vi "Ejercicio_6_Queued.vi"() -> ()   [LabVIEW 2020]
panel:
  out "Waveform Chart":dbl(graph)
  in  "stop":bool
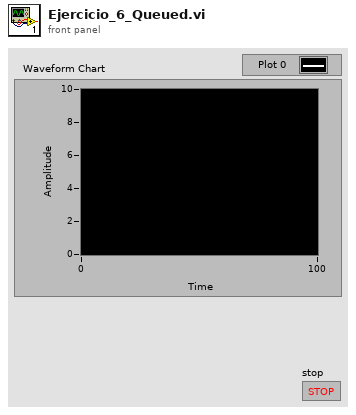
[diagram p1: front panel]
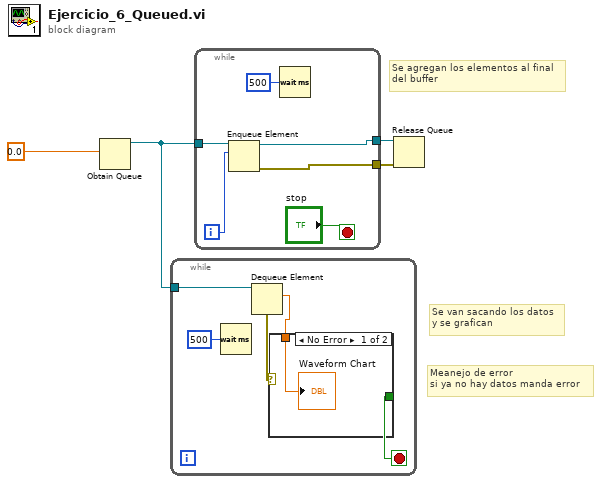
[diagram p0: block diagram]
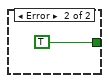
[diagram p2: hidden frame]
diagram:
  # "Se agregan los elementos al final\ndel buffer"
  # "Meanejo de error\nsi ya no hay datos manda error"
  # "Se van sacando los datos\ny se grafican"
  n1 = Obtain Queue(element data type=0.0) -> (queue out=w3:refnum<queue>)  [unwired: 4 in, 2 out]
  n2 = while {
    tunnel: w3 -> [w9]
    stop <- w6 stop-if-true
    n3 = Wait (ms)(milliseconds to wait=u32 500) -> ()  [unwired: 1 out]
    n4 = Dequeue Element(queue=w9) -> (element=w5:dbl, error out=w7:errorcluster)  [unwired: 2 in, 2 out]
    n5 = case shown="No Error" w7 {
      tunnel: [_ TRUE] -> w6
      tunnel: w5 -> [w10 _]
      frame No Error {
        "Waveform Chart" <- w10
      }
      frame Error {
      }
    }
  }
  n6 = while {
    tunnel: w3 -> [w17]
    tunnel: [w13] -> w4
    tunnel: [w15] -> w1
    i -> [w12]
    stop <- "stop" stop-if-true
    n7 = Enqueue Element(queue=w17, element=w12) -> (queue out=w13:refnum<queue>, error out=w15:errorcluster)  [unwired: 2 in, 1 out]
    n8 = Wait (ms)(milliseconds to wait=u32 500) -> ()  [unwired: 1 out]
  }
  n9 = Release Queue(queue=w4, error in (no error)=w1) -> ()  [unwired: 1 in, 3 out]
